vi "Get Channels For Measurement.vi"(8 "error in (no error)":errorcluster, 10 "property name":string, 11 "Node Ptr in":T1 format="%.0x") -> (0 "error out":errorcluster, 2 "rios and channels":T2(array[cluster]), 3 "Node Ptr out":T1 format="%.0x")   [LabVIEW 2017, in "Engine Simulation Toolkit System Explorer.lvlib"]
uses:
  Engine Simulation Toolkit System Explorer.lvlib
  <vilib>/NI Veristand/Custom Device API/Custom Device Item Ref.ctl
  <vilib>/NI Veristand/Custom Device API/Custom Device API.lvlib
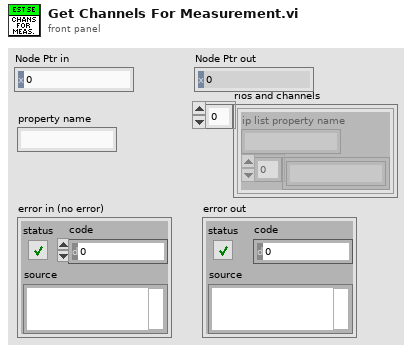
[diagram p1: front panel]
types:
  T1 = typedef "Custom Device API.lvlib/Custom Device Item Ref.ctl" = u64
  T2 = cluster{"ip list property name":string, string[]}[]
  T3 = typedef "Custom Device API.lvlib/Custom Device Item Info.ctl" = cluster{"Name":string, "Is Channel":bool, "GUID":string, "Is Waveform":bool}
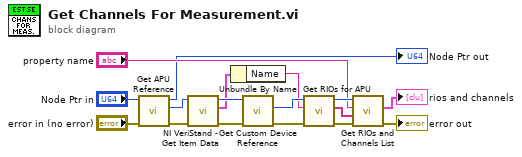
[diagram p0: block diagram]
diagram:
  n1 = call "Get APU Reference.vi"("error in (no error)"="error in (no error)", "Item Ref in"="Node Ptr in") -> ("error out"=w10:errorcluster, "APU Ref"=w11:T1, "Item Ref out"=→"Node Ptr out":T1)  [unwired: 7 in]
  n2 = call <vilib>:"NI VeriStand - Get Item Data.vi"("error in (no error)"=w10, "Item Ref in"=w11) -> ("error out"=w14:errorcluster, "Item Info"=w12:T3, "Item Ref out"=w16:T1)  [unwired: 6 in, 1 out]
  n3 = Unbundle By Name(w12) -> ("Name"=w13:string)
  n4 = call "Get Custom Device Reference.vi"("error in (no error)"=w14, "Item Ref in"=w16) -> ("error out"=w15:errorcluster, "Custom Device Ref"=w17:T1)  [unwired: 7 in, 1 out]
  n5 = call "Get RIOs for APU.vi"("error in (no error)"=w15, "APU name"=w13, "Item Ref in"=w17) -> ("error out"=w7:errorcluster, "RIO Addresses"=w9:string[], "Item Ref out"=w8:T1)  [unwired: 6 in]
  n6 = call "Get RIOs and Channels List.vi"("error in (no error)"=w7, "rio names"=w9, "ip list property name"="property name", "Item Ref in"=w8) -> ("error out"=→"error out":errorcluster, "rios and channels"=→"rios and channels":T2)  [unwired: 5 in, 1 out]
